vi "Periodic Tasks.vi"(8 "error in":errorcluster) -> ()   [LabVIEW 2013]
doc: "This VI runs in parallel to other tasks. It can contain as many user-defined periodic loops as you need. These can carry out PID or other sorts of timed response."
uses:
  Shooter States.ctl
  <vilib>/Rock Robotics/SystemInterfaces/Utilities/FPGA_UtilitiesLED Source.ctl
  <vilib>/Rock Robotics/SystemInterfaces/Utilities/FPGA_UtilitiesLED State.ctl
  <vilib>/Rock Robotics/WPI/Solenoid/WPI_SolenoidValue.ctl
  Robot Global Data.vi
  <vilib>/Rock Robotics/WPI/Compressor/WPI_CompressorGetSetRefNum.vi
  <vilib>/Rock Robotics/WPI/Joystick/WPI_JoystickGetSetRefNum.vi
  <vilib>/Rock Robotics/WPI/Solenoid/WPI_SolenoidSetEnum.vi
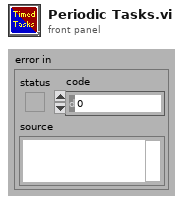
[diagram p1: front panel]
types:
  T1 = typedef "Shooter States.ctl" = enum16{"Init", "Latch set", "shooter set", "release", "reset"}
  T2 = typedef "FPGA_UtilitiesLED State.ctl" = enum16{"Off", "On", "Toggle"}
  T3 = typedef "FPGA_UtilitiesLED Source.ctl" = enum16{"User LED", "FPGA LED"}
  T4 = typedef "WPI_CompressorDevRef.ctl" = cluster{"DevStatus":errorcluster, "DigitalInputDevRef":T5, "RelayDevRef":T8}
  T5 = typedef "WPI_DigitalInputDevRef.ctl" = cluster{"DevStatus":errorcluster, "DIO Channel":T6, "Digital Module":T7}
  T6 = typedef "FPGA_DIOChannel.ctl" = enum8{"DIO 1", "DIO 2", "DIO 3", "DIO 4", "DIO 5", "DIO 6", "DIO 7", "DIO 8", "DIO 9", "DIO 10", "DIO 11", "DIO 12", "DIO 13", "DIO 14", "Invalid"}
  T7 = typedef "FPGA_TypedefDigitalModule.ctl" = enum16{"Digital Module 1", "Digital Module 2"}
  T8 = typedef "WPI_RelayDevRef.ctl" = cluster{"DevStatus":errorcluster, "Relay Channel":T9, "Digital Module":T7, "Relay Direction":T10}
  T9 = typedef "FPGA_DIORelayChannel.ctl" = enum8{"Relay 1", "Relay 2", "Relay 3", "Relay 4", "Relay 5", "Relay 6", "Relay 7", "Relay 8", "Invalid"}
  T10 = typedef "WPI_RelayDirection.ctl" = enum16{"Both directions", "Forward only", "Reverse only"}
  T11 = typedef "WPI_SolenoidDevRef.ctl" = cluster{"DevStatus":errorcluster, "Solenoid Module":T12, "Forward Solenoid Channel":T13, "Reverse Solenoid Channel":T13}
  T12 = typedef "FPGA_TypedefSolenoidModule.ctl" = enum16{"Solenoid Module 1", "Solenoid Module 2"}
  T13 = typedef "WPI_SolenoidChannel.ctl" = enum8{"Solenoid 1", "Solenoid 2", "Solenoid 3", "Solenoid 4", "Solenoid 5", "Solenoid 6", "Solenoid 7", "Solenoid 8", "Invalid"}
  T14 = typedef "WPI_JoystickDevRef.ctl" = cluster{"Device":T15}
  T15 = typedef "WPI_JoystickDeviceEnum.ctl" = enum16{"USB 1", "USB 2", "USB 3", "USB 4", "Kinect 1", "Kinect 2"}
  T16 = typedef "WPI_SolenoidValue.ctl" = enum16{"Off", "On", "Forward", "Reverse"}
  T17 = typedef "WPI_JoystickButtonState.ctl" = cluster{"Button 1":bool, "Button 2":bool, "Button 3":bool, "Button 4":bool, "Button 5":bool, "Button 6":bool, "Button 7":bool, "Button 8":bool, "Button 9":bool, "Button 10":bool, "Button 11":bool, "Button 12":bool}
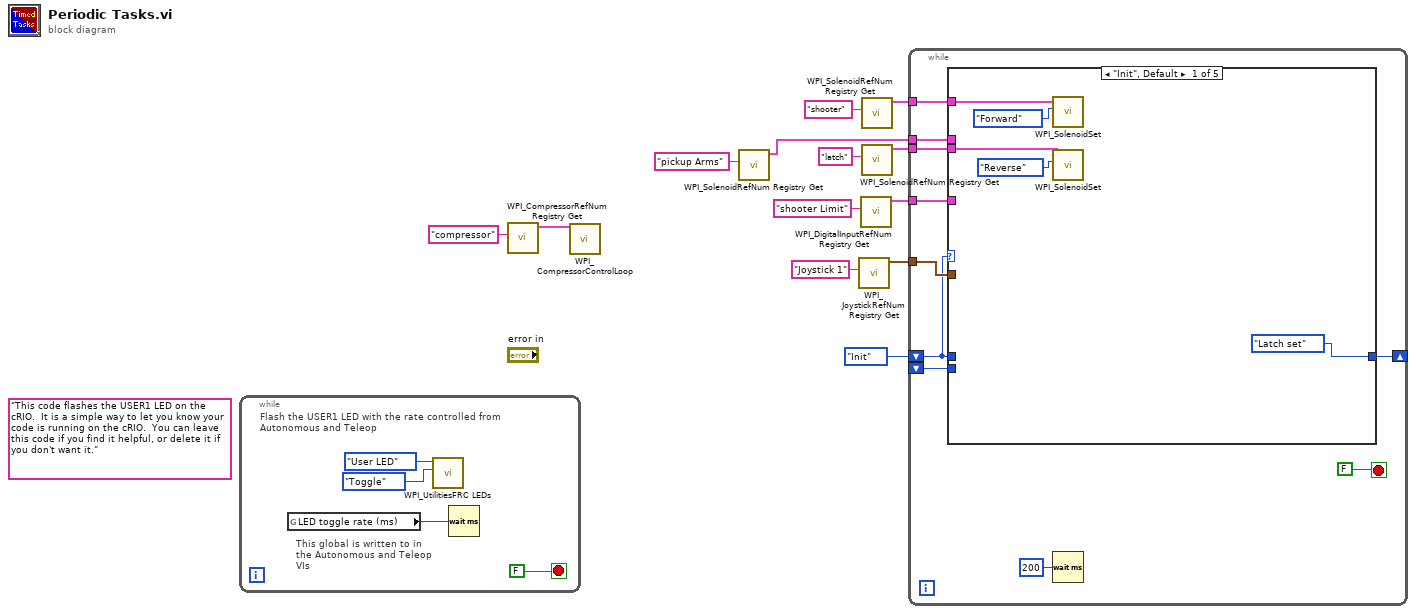
[diagram p0: block diagram]
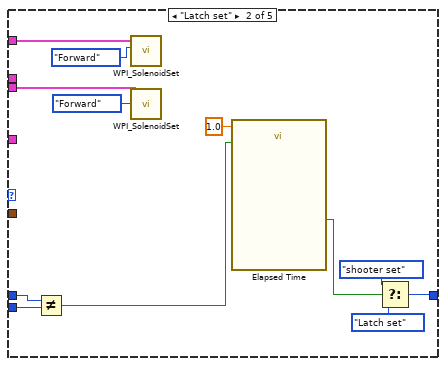
[diagram p2: hidden frame]
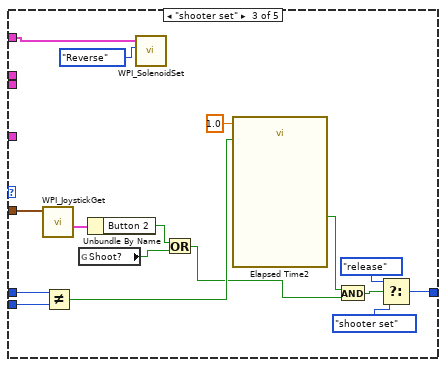
[diagram p3: hidden frame]
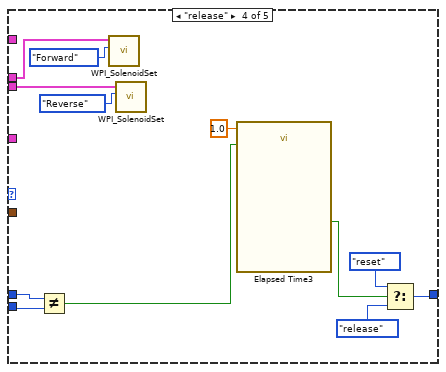
[diagram p4: hidden frame]
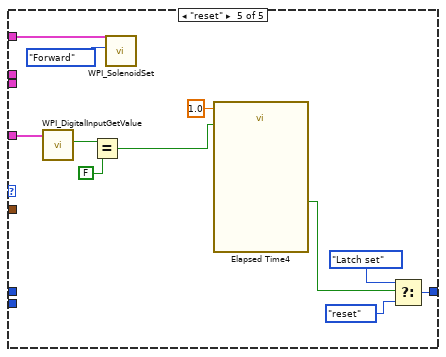
[diagram p5: hidden frame]
diagram:
  w5 = Shooter_States."Init"
  (unwired) "This code flashes the USER1 LED on the cRIO.  It is a simple way to let you know your code is running on the cRIO.  You can leave this code if you find it helpful, or delete it if you don't want it."
  n1 = while {
    stop <- FALSE stop-if-true
    # "This global is written to in the Autonomous and Teleop VIs"
    # "Flash the USER1 LED with the rate controlled from Autonomous and Teleop"
    n2 = global read "Robot Global Data.vi" "LED toggle rate (ms)"() -> (w14:u32)
    n3 = call <vilib>:"WPI_UtilitiesFRC LEDs.vi"("State"=FPGA_UtilitiesLED_State."Toggle", "LED Type"=FPGA_UtilitiesLED_Source."User LED") -> ()  [unwired: 1 in, 9 out]
    n4 = Wait (ms)(milliseconds to wait=w14) -> ()  [unwired: 1 out]
  }
  n5 = call <vilib>:"WPI_CompressorRefNum Registry Get.vi"("refnum name"="compressor") -> ("CompressorDevRef"=w3:T4)  [unwired: 9 in, 1 out]
  n6 = call <vilib>:"WPI_CompressorControlLoop.vi"("CompressorDevRef"=w3) -> ()  [unwired: 11 in]
  n7 = call <vilib>:"WPI_SolenoidRefNum Registry Get.vi"("refnum name"="pickup Arms") -> ("SolenoidDevRef"=w1:T11)  [unwired: 9 in, 1 out]
  n8 = call <vilib>:"WPI_JoystickRefNum Registry Get.vi"("refnum name"="Joystick 1") -> ("JoystickDevRef"=w6:T14)  [unwired: 9 in, 1 out]
  n9 = call <vilib>:"WPI_DigitalInputRefNum Registry Get.vi"("refnum name"="shooter Limit") -> ("DigitalInputDevRef"=w8:T5)  [unwired: 9 in, 1 out]
  n10 = call <vilib>:"WPI_SolenoidRefNum Registry Get.vi"("refnum name"="shooter") -> ("SolenoidDevRef"=w11:T11)  [unwired: 9 in, 1 out]
  n11 = call <vilib>:"WPI_SolenoidRefNum Registry Get.vi"("refnum name"="latch") -> ("SolenoidDevRef"=w10:T11)  [unwired: 9 in, 1 out]
  n12 = while {
    shift-right: [w24] -> _
    shift-left: w5 -> [w20]
    tunnel: w11 -> [w26]
    tunnel: w10 -> [w25]
    tunnel: w8 -> [w19]
    tunnel: w6 -> [w22]
    shift-left: w5 -> [w23]
    tunnel: w1 -> [w18]
    stop <- FALSE stop-if-true
    n13 = case shown="\"Init\", Default" w20 {
      tunnel: w26 -> [w32 w42 w59 _ w79]
      tunnel: w25 -> [w31 w41 _ w67 _]
      tunnel: [Shooter_States."Latch set" w39 w55 w70 w80] -> w24
      tunnel: w23 -> [_ w35 w53 w65 _]
      tunnel: w20 -> [_ w34 w54 w66 _]
      tunnel: w22 -> [_ _ w51 _ _]
      tunnel: w19 -> [_ _ _ _ w78]
      tunnel: w18 -> [_ _ _ w62 _]
      frame "Init", Default {
        n14 = call-poly <vilib>:"WPI_SolenoidSet.vi"("Value"=WPI_SolenoidValue."Forward", "SolenoidDevRef"=w32) -> ()  [unwired: 8 in, 2 out]
        n15 = call-poly <vilib>:"WPI_SolenoidSet.vi"("Value"=WPI_SolenoidValue."Reverse", "SolenoidDevRef"=w31) -> ()  [unwired: 8 in, 2 out]
      }
      frame "Latch set" {
        n16 = Not Equal?(x=w34, y=w35) -> (x != y?=w33:bool)
        n17 = call-poly <vilib>:"WPI_SolenoidSet.vi"("Value"=WPI_SolenoidValue."Forward", "SolenoidDevRef"=w42) -> ()  [unwired: 8 in, 2 out]
        n18 = call-poly <vilib>:"WPI_SolenoidSet.vi"("Value"=WPI_SolenoidValue."Forward", "SolenoidDevRef"=w41) -> ()  [unwired: 8 in, 2 out]
        n19 = call "Elapsed Time"("Time Target (s)"=1.0, "Reset"=w33) -> ("Time has Elapsed"=w38:bool)  [unwired: 10 in, 7 out]
        n20 = Select(t=Shooter_States."shooter set", s=w38, f=Shooter_States."Latch set") -> (s? t:f=w39:T1)
      }
      frame "shooter set" {
        n21 = call <vilib>:"WPI_JoystickGet.vi"("JoystickDevRef"=w51) -> ("Buttons"=w50:T17)  [unwired: 4 in, 2 out]
        n22 = Not Equal?(x=w54, y=w53) -> (x != y?=w52:bool)
        n23 = global read "Robot Global Data.vi" "Shoot?"() -> (w45:bool)
        n24 = Unbundle By Name(w50) -> ("Button 2"=w47:bool)
        n25 = call-poly <vilib>:"WPI_SolenoidSet.vi"("Value"=WPI_SolenoidValue."Reverse", "SolenoidDevRef"=w59) -> ()  [unwired: 8 in, 2 out]
        n26 = Or(x=w47, y=w45) -> (x .or. y?=w46:bool)
        n27 = call "Elapsed Time2"("Time Target (s)"=1.0, "Reset"=w52) -> ("Time has Elapsed"=w48:bool)  [unwired: 10 in, 7 out]
        n28 = And(x=w48, y=w46) -> (x .and. y?=w49:bool)
        n29 = Select(t=Shooter_States."release", s=w49, f=Shooter_States."shooter set") -> (s? t:f=w55:T1)
      }
      frame "release" {
        n30 = Not Equal?(x=w66, y=w65) -> (x != y?=w64:bool)
        n31 = call-poly <vilib>:"WPI_SolenoidSet.vi"("Value"=WPI_SolenoidValue."Forward", "SolenoidDevRef"=w62) -> ()  [unwired: 8 in, 2 out]
        n32 = call-poly <vilib>:"WPI_SolenoidSet.vi"("Value"=WPI_SolenoidValue."Reverse", "SolenoidDevRef"=w67) -> ()  [unwired: 8 in, 2 out]
        n33 = call "Elapsed Time3"("Time Target (s)"=1.0, "Reset"=w64) -> ("Time has Elapsed"=w69:bool)  [unwired: 10 in, 7 out]
        n34 = Select(t=Shooter_States."reset", s=w69, f=Shooter_States."release") -> (s? t:f=w70:T1)
      }
      frame "reset" {
        n35 = call <vilib>:"WPI_DigitalInputGetValue.vi"("DigitalInputDevRef"=w78) -> ("Value"=w75:bool)  [unwired: 8 in, 2 out]
        n36 = Equal?(x=w75, y=FALSE) -> (x = y?=w73:bool)
        n37 = call-poly <vilib>:"WPI_SolenoidSet.vi"("Value"=WPI_SolenoidValue."Forward", "SolenoidDevRef"=w79) -> ()  [unwired: 8 in, 2 out]
        n38 = call "Elapsed Time4"("Time Target (s)"=1.0, "Reset"=w73) -> ("Time has Elapsed"=w76:bool)  [unwired: 10 in, 7 out]
        n39 = Select(t=Shooter_States."Latch set", s=w76, f=Shooter_States."reset") -> (s? t:f=w80:T1)
      }
    }
    n40 = Wait (ms)(milliseconds to wait=u32 200) -> ()  [unwired: 1 out]
  }
